vi "_Subscribe.vi"(8 "error in (no error)":errorcluster, 10 "Subscription":T1, 11 "Loop Data In":T2) -> (0 "error out":errorcluster, 3 "Loop Data":T2)   [LabVIEW 2020, in "Vecto.lvlib" / "RemoteDataService.lvclass"]
uses:
  RemoteDataService.lvclass
  Loop Data.ctl
  SequenceCountService/SequenceCountService.lvclass
  ChannelService/ChannelService.lvclass
  Published Group.ctl
  Packet.ctl
  <vilib>/IlluminatedG/IG Protoc/LV-Proto/Message/Message.lvclass
  Subscription.ctl
  Subscription Info.ctl
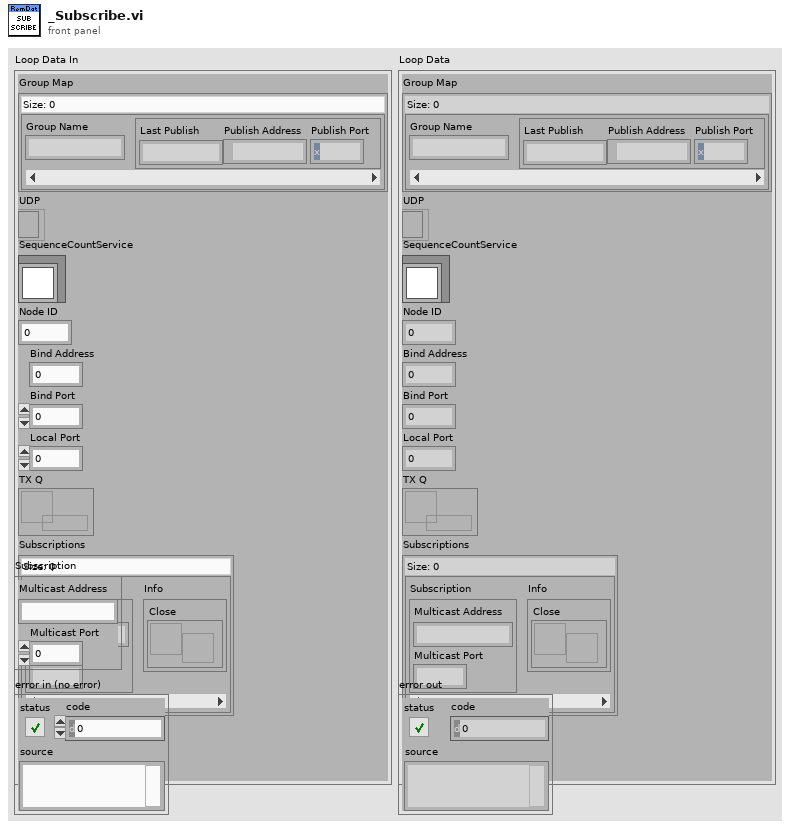
[diagram p1: front panel]
types:
  T1 = typedef "Vecto.lvlib/RemoteDataService.lvclass/Subscription.ctl" = cluster{"Multicast Address":string, "Multicast Port":u16}
  T2 = typedef "Vecto.lvlib/RemoteDataService.lvclass/Loop Data.ctl" = cluster{"Group Map":map{string, T3}, "UDP":refnum<k16>, "SequenceCountService":refnum<class "SequenceCountService.lvclass">, "Node ID":u32, "Bind Address":u32, "Bind Port":u16, "Local Port":u16, "TX Q":refnum<queue>, "Subscriptions":map{T1, T4}, "ChannelService":refnum<class "ChannelService.lvclass">}
  T3 = typedef "Vecto.lvlib/RemoteDataService.lvclass/Published Group.ctl" = cluster{"Last Publish":dbl, "Publish Address":u32, "Publish Port":u16}
  T4 = typedef "Vecto.lvlib/RemoteDataService.lvclass/Subscription Info.ctl" = cluster{"Close":refnum<user-event>}
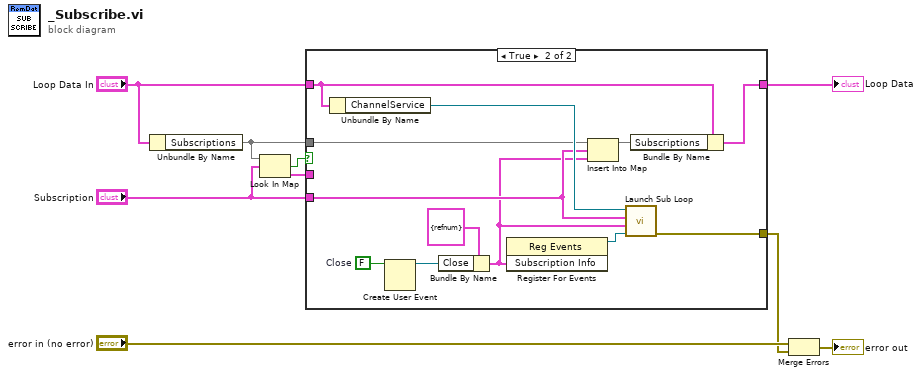
[diagram p0: block diagram]
diagram:
  n1 = Unbundle By Name("Loop Data In") -> ("Subscriptions"=w8:map{T1, T4})
  n2 = Look In Map(map=w8, key="Subscription") -> (key not found?=w9:bool, value=w7:T4)  [unwired: 1 in]
  n3 = case shown="True" w9 {
    tunnel: w8 -> [_ w17]
    tunnel: w7 -> [_ _]
    tunnel: "Subscription" -> [_ w16]
    tunnel: "Loop Data In" -> [w10 w14]
    tunnel: [w10 w12] -> w3
    tunnel: [_ w11] -> w1
    frame False {
      # "Already subscribed to endpoint"
    }
    frame True {
      w22 = FALSE  # Close
      n4 = Unbundle By Name(w14) -> ("ChannelService"=w18:refnum<class "ChannelService.lvclass">)
      n5 = Create User Event(user event datatype=w22) -> (user event=w20:refnum<user-event>)  [unwired: 1 in, 1 out]
      n6 = Bundle By Name(cluster=T4 {"Close"=refnum} ("Subscription Info"), "Close"=w20) -> (w15:T4)
      n7 = register-events(w15) -> (reference out=w19:refnum<event-registration>)  [unwired: 2 in, 1 out]
      n8 = Insert Into Map(map in=w17, key=w16, value=w15) -> (map out=w13:map{T1, T4})  [unwired: 2 out]
      n9 = call "Launch Sub Loop.vi"("Event Reg"=w19, "Subscription Info"=w15, "Subscription"=w16, "ChannelService"=w18) -> ("error out"=w11:errorcluster)  [unwired: 7 in]
      n10 = Bundle By Name(cluster=w14, "Subscriptions"=w13) -> (w12:T2)
    }
  }
  "Loop Data" <- w3
  n11 = Merge Errors("error in (no error)", w1) -> (→"error out":errorcluster)
